vi "main(Test DQMH modules).vi"() -> ()   [LabVIEW 2018, in "Application.lvlib"] (continued)
      tunnel: w245 -> [w281 _ _ _ w1278 w1403 _ w1480 _ _ _ _ _ _ _ _ _ _ _ _ _ _ _ _ _ _ _ _ _ _ _ _ _ _ _ _ _ _ _ _ _ _ _ _ w2433 _ _ _ _ _ _ _ _ _ _ _ _ _ _ _ _ _ _ _ _ _ _ _ _ _ _ _ _ _ _ _ _ _ _ _ _ _ _ _ _ _ _ _ _ _ _ _ _ _ _ _ _ _ _ _ _ _ _ _ _ _ _ _ _ _ _ _ _ _ _ _ _ _ _ _ _ _ _ _ _ _ _ _ _ _ _ _ _ _ _ _ _ _ _ _ _ _ _ _ _ _ _ _ _ _ _ _ _ _ _ _ _ _ _ _ _ _ _ _ _ _ w9912 w10010 w10108 w10208 w10305 w10404 w10503 w10602 w10701 w10800 w10899 w10998 w11097 w11196 w11295 w11394 w11493 w11592 w11691 w11790 w11889 w11988 w12087 w12186 w12285 w12384 w12483 w12582 w12681 w12780 w12879 w12978 w13077 w13176 w13275 w13374 w13473 w13572 w13671 w13770 w13869 w13968 w14067 w14166 w14265 w14364 w14463 w14562 w14661 w14760 w14859 w14958 w15057 w15156 w15255 w15354 w15453 w15552 w15651 w15750]
      tunnel: [w274 w1237 w1249 w1259 w1277 w1409 w1450 w1490 w1515 w1531 w1542 w1553 w1568 w1583 w1598 w1613 w1627 w1651 w1680 w1710 w1766 w1803 w1825 w1848 w1870 w1903 w1921 w1939 w1957 w1989 w2017 w2042 w2070 w2103 w2122 w2144 w2177 w2194 w2219 w2247 w2279 w2309 w2354 w2387 w2432 w2497 w2573 w2648 w2723 w2798 w2873 w2934 w3037 w3113 w3187 w3271 w3353 w3435 w3517 w3599 w3681 w3763 w3845 w3927 w4009 w4091 w4174 w4257 w4340 w4423 w4506 w4571 w4690 w4773 w4856 w4939 w5023 w5107 w5191 w5275 w5359 w5443 w5527 w5611 w5695 w5779 w5864 w5949 w6034 w6119 w6204 w6289 w6374 w6459 w6544 w6629 w6715 w6801 w6887 w6973 w7059 w7145 w7231 w7317 w7403 w7449 w7491 w7531 w7572 w7613 w7654 w7695 w7736 w7777 w7818 w7859 w7900 w7941 w7982 w8023 w8065 w8105 w8146 w8187 w8228 w8270 w8310 w8352 w8392 w8433 w8475 w8515 w8556 w8597 w8638 w8679 w8720 w8761 w8803 w8843 w8884 w8925 w8967 w9008 w9048 w9089 w9130 w9171 w9212 w9253 w9294 w9335 w9376 w9417 w9458 w9499 w9540 w9581 w9622 w9663 w9704 w9745 w9786 w9827 w9868 w9903 1 ("DUT channel (1-11)") 1 ("DUT channel (1-11)") 1 ("DUT channel (1-11)") 1 ("DUT channel (1-11)") 1 ("DUT channel (1-11)") 1 ("DUT channel (1-11)") 2 ("DUT channel (1-11)") 2 ("DUT channel (1-11)") 2 ("DUT channel (1-11)") 2 ("DUT channel (1-11)") 2 ("DUT channel (1-11)") 2 ("DUT channel (1-11)") 3 ("DUT channel (1-11)") 3 ("DUT channel (1-11)") 3 ("DUT channel (1-11)") 3 ("DUT channel (1-11)") 3 ("DUT channel (1-11)") 3 ("DUT channel (1-11)") 4 ("DUT channel (1-11)") 4 ("DUT channel (1-11)") 4 ("DUT channel (1-11)") 4 ("DUT channel (1-11)") 4 ("DUT channel (1-11)") 4 ("DUT channel (1-11)") 5 ("DUT channel (1-11)") 5 ("DUT channel (1-11)") 5 ("DUT channel (1-11)") 5 ("DUT channel (1-11)") 5 ("DUT channel (1-11)") 5 ("DUT channel (1-11)") 6 ("DUT channel (1-11)") 6 ("DUT channel (1-11)") 6 ("DUT channel (1-11)") 6 ("DUT channel (1-11)") 6 ("DUT channel (1-11)") 6 ("DUT channel (1-11)") 7 ("DUT channel (1-11)") 7 ("DUT channel (1-11)") 7 ("DUT channel (1-11)") 7 ("DUT channel (1-11)") 7 ("DUT channel (1-11)") 7 ("DUT channel (1-11)") 8 ("DUT channel (1-11)") 8 ("DUT channel (1-11)") 8 ("DUT channel (1-11)") 8 ("DUT channel (1-11)") 8 ("DUT channel (1-11)") 8 ("DUT channel (1-11)") 9 ("DUT channel (1-11)") 9 ("DUT channel (1-11)") 9 ("DUT channel (1-11)") 9 ("DUT channel (1-11)") 9 ("DUT channel (1-11)") 9 ("DUT channel (1-11)") 10 ("DUT channel (1-11)") 10 ("DUT channel (1-11)") 10 ("DUT channel (1-11)") 10 ("DUT channel (1-11)") 10 ("DUT channel (1-11)") 10 ("DUT channel (1-11)")] -> w244
      tunnel: w243 -> [w275 w1237 w1249 w1259 w1277 w1409 w1450 w1490 w1515 w1531 w1542 w1553 w1568 w1583 w1598 w1613 w1627 w1651 w1680 w1710 w1766 w1803 w1825 w1848 w1870 w1903 w1921 w1939 w1957 w1989 w2017 w2042 w2070 w2103 w2122 w2144 w2177 w2194 w2219 w2247 w2279 w2309 w2354 w2387 w2432 _ _ _ _ _ _ _ _ _ _ _ _ _ _ _ _ _ _ _ _ _ _ _ _ _ _ _ _ _ _ _ _ _ _ _ _ _ _ _ _ _ _ _ _ _ _ _ _ _ _ _ _ _ _ _ _ _ _ _ _ w7449 w7491 w7531 w7572 w7613 w7654 w7695 w7736 w7777 w7818 w7859 w7900 w7941 w7982 w8023 w8065 w8105 w8146 w8187 w8228 w8270 w8310 w8352 w8392 w8433 w8475 w8515 w8556 w8597 w8638 w8679 w8720 w8761 w8803 w8843 w8884 w8925 w8967 w9008 w9048 w9089 w9130 w9171 w9212 w9253 w9294 w9335 w9376 w9417 w9458 w9499 w9540 w9581 w9622 w9663 w9704 w9745 w9786 w9827 w9868 w9903 _ _ _ _ _ _ _ _ _ _ _ _ _ _ _ _ _ _ _ _ _ _ _ _ _ _ _ _ _ _ _ _ _ _ _ _ _ _ _ _ _ _ _ _ _ _ _ _ _ _ _ _ _ _ _ _ _ _ _ _]
      tunnel: [w272 w1236 w1248 w1258 w1279 w1397 w1449 w1489 w1514 w1530 w1541 w1552 w1567 w1582 w1597 w1612 w1626 w1650 w1679 w1709 w1765 w1802 w1824 w1847 w1869 w1902 w1920 w1938 w1956 w1988 w2016 w2041 w2069 w2102 w2121 w2143 w2176 w2193 w2218 w2250 w2278 w2308 w2353 w2378 w2431 w2481 w2572 w2647 w2722 w2797 w2872 w2933 w3036 w3112 w3186 w3270 w3352 w3434 w3516 w3598 w3680 w3762 w3844 w3926 w4008 w4090 w4173 w4256 w4339 w4422 w4505 w4570 w4689 w4772 w4855 w4938 w5022 w5106 w5190 w5274 w5358 w5442 w5526 w5610 w5694 w5778 w5863 w5948 w6033 w6118 w6203 w6288 w6373 w6458 w6543 w6628 w6714 w6800 w6886 w6972 w7058 w7144 w7230 w7316 w7402 w7445 w7487 w7527 w7568 w7609 w7653 w7691 w7732 w7773 w7814 w7855 w7896 w7937 w7978 w8019 w8061 w8101 w8145 w8183 w8224 w8266 w8306 w8348 w8388 w8429 w8471 w8511 w8552 w8593 w8634 w8675 w8716 w8757 w8799 w8839 w8880 w8921 w8963 w9004 w9044 w9085 w9126 w9167 w9208 w9249 w9290 w9331 w9372 w9413 w9454 w9495 w9536 w9577 w9618 w9660 w9700 w9741 w9782 w9823 w9864 w9902 w9911 w10009 w10107 w10207 w10304 w10403 w10502 w10601 w10700 w10799 w10898 w10997 w11096 w11195 w11294 w11393 w11492 w11591 w11690 w11789 w11888 w11987 w12086 w12185 w12284 w12383 w12482 w12581 w12680 w12779 w12878 w12977 w13076 w13175 w13274 w13373 w13472 w13571 w13670 w13769 w13868 w13967 w14066 w14165 w14264 w14363 w14462 w14561 w14660 w14759 w14858 w14957 w15056 w15155 w15254 w15353 w15452 w15551 w15650 w15749] -> w242
      tunnel: w241 -> [w273 w1236 w1248 w1258 w1279 w1397 w1449 w1489 w1514 w1530 w1541 w1552 w1567 w1582 w1597 w1612 w1626 w1650 w1679 w1709 w1765 w1802 w1824 w1847 w1869 w1902 w1920 w1938 w1956 w1988 w2016 w2041 w2069 w2102 w2121 w2143 w2176 w2193 w2218 w2250 w2278 w2308 w2353 w2378 w2431 w2481 w2572 w2647 w2722 w2797 w2872 w2933 w3036 w3112 w3186 w3270 w3352 w3434 w3516 w3598 w3680 w3762 w3844 w3926 w4008 w4090 w4173 w4256 w4339 w4422 w4505 w4570 w4689 w4772 w4855 w4938 w5022 w5106 w5190 w5274 w5358 w5442 w5526 w5610 w5694 w5778 w5863 w5948 w6033 w6118 w6203 w6288 w6373 w6458 w6543 w6628 w6714 w6800 w6886 w6972 w7058 w7144 w7230 w7316 w7402 _ _ _ _ _ _ _ _ _ _ _ _ _ _ _ _ _ _ _ _ _ _ _ _ _ _ _ _ _ _ _ _ _ _ _ _ _ _ _ _ _ _ _ _ _ _ _ _ _ _ _ _ _ _ _ _ _ _ _ _ w9902 _ _ _ _ _ _ _ _ _ _ _ _ _ _ _ _ _ _ _ _ _ _ _ _ _ _ _ _ _ _ _ _ _ _ _ _ _ _ _ _ _ _ _ _ _ _ _ _ _ _ _ _ _ _ _ _ _ _ _ _]
      tunnel: w238 -> [w280 _ _ _ _ _ _ _ _ _ _ _ _ _ _ _ _ _ _ _ _ _ _ _ _ _ _ _ _ _ _ _ _ w2097 _ _ _ _ _ _ _ _ _ _ _ _ _ _ _ _ _ _ _ _ _ _ _ _ _ _ _ _ _ _ _ _ _ _ _ _ _ _ _ _ _ _ _ _ _ _ _ _ _ _ _ _ _ _ _ _ _ _ _ _ _ _ _ _ _ _ _ _ _ _ _ _ _ _ _ _ _ _ _ _ _ _ _ _ _ _ _ _ _ _ _ _ _ _ _ _ _ _ _ _ _ _ _ _ _ _ _ _ _ _ _ _ _ _ _ _ _ _ _ _ _ _ _ _ _ _ _ _ _ _ _ _ _ _ _ _ _ _ _ _ _ _ _ _ _ _ _ _ _ _ _ _ _ _ _ _ _ _ _ _ _ _ _ _ _ _ _ _ _ _ _ _ _ _ _ _ _ _ _ _ _ _ _ _ _ _ _ _ _ _ _ _]
      tunnel: [_ _ _ _ _ _ _ _ _ _ _ _ _ _ _ _ _ _ _ _ _ _ _ _ _ _ _ _ _ _ _ _ _ _ _ _ _ _ _ _ _ _ _ TRUE _ _ _ _ _ _ _ _ _ _ _ _ _ _ _ _ _ _ _ _ _ _ _ _ _ _ _ _ _ _ _ _ _ _ _ _ _ _ _ _ _ _ _ _ _ _ _ _ _ _ _ _ _ _ _ _ _ _ _ _ _ _ _ _ _ _ _ _ _ _ _ _ _ _ _ _ _ _ _ _ _ _ _ _ _ _ _ _ _ _ _ _ _ _ _ _ _ _ _ _ _ _ _ _ _ _ _ _ _ _ _ _ _ _ _ _ _ _ _ _ _ _ _ _ _ _ _ _ _ _ _ _ _ _ _ _ _ _ _ _ _ _ _ _ _ _ _ _ _ _ _ _ _ _ _ _ _ _ _ _ _ _ _ _ _ _ _ _ _ _ _ _ _ _ _ _ _ _ _ _ _ _] -> w237
      tunnel: [w276 "Waiting for JIG lock" w1242 w1254 w1275 w1407 w1422 w1481 w1513 w1529 w1540 w1551 w1566 w1581 w1596 w1611 w1624 w1646 w1678 "Initialize Apps" w1747 w1798 w1820 w1843 w1864 w1897 w1915 w1933 w1951 w1978 w2011 w2038 w2066 w2093 "HV-60D ready!!!!!!!!!!!!!!!!" w2138 w2173 w2188 w2211 w2244 w2274 w2303 w2346 w2380 "Shorted Circuit Test" "Test Channel 1" "Test Channel 2" "Test Channel 3" "Test Channel 4" "Test Channel 5" "Test Channel 6" "Test Channel 7" "Test Channel 8" "Test Channel 9" "Test Channel 10" "Test Channel 10A" "Test Channel 1A" "Test Channel 2A" "Test Channel 3A" "Test Channel 4A" "Test Channel 5A" "Test Channel 6A" "Test Channel 7A" "Test Channel 8A" "Test Channel 9A" "Test Channel 10B" "Test Channel 1B" "Test Channel 2B" "Test Channel 3B" "Test Channel 4B" "Test Channel 5B" "Test Channel 6B" "Test Channel 7B" "Test Channel 8B" "Test Channel 9B" "Test Channel 10C" "Test Channel 1C" "Test Channel 2C" "Test Channel 3C" "Test Channel 4C" "Test Channel 5C" "Test Channel 6C" "Test Channel 7C" "Test Channel 8C" "Test Channel 9C" "Test Channel 10D" "Test Channel 1D" "Test Channel 2D" "Test Channel 3D" "Test Channel 4D" "Test Channel 5D" "Test Channel 6D" "Test Channel 7D" "Test Channel 8D" "Test Channel 9D" "Test Channel 10E" "Test Channel 1E" "Test Channel 2E" "Test Channel 3E" "Test Channel 4E" "Test Channel 5E" "Test Channel 6E" "Test Channel 7E" "Test Channel 8E" "Test Channel 9E" w7447 w7490 w7530 w7571 w7612 w7652 w7694 w7735 w7776 w7817 w7858 w7899 w7940 w7981 w8022 w8064 w8104 w8144 w8186 w8227 w8269 w8309 w8351 w8391 w8432 w8474 w8514 w8555 w8596 w8637 w8678 w8719 w8760 w8802 w8842 w8883 w8924 w8966 w9007 w9047 w9088 w9129 w9170 w9211 w9252 w9293 w9334 w9375 w9416 w9457 w9498 w9539 w9580 w9621 w9662 w9703 w9744 w9785 w9826 w9867 w9901 w9916 w10014 w10112 w10210 w10309 w10408 w10507 w10606 w10705 w10804 w10903 w11002 w11101 w11200 w11299 w11398 w11497 w11596 w11695 w11794 w11893 w11992 w12091 w12190 w12289 w12388 w12487 w12586 w12685 w12784 w12883 w12982 w13081 w13180 w13279 w13378 w13477 w13576 w13675 w13774 w13873 w13972 w14071 w14170 w14269 w14368 w14467 w14566 w14665 w14764 w14863 w14962 w15061 w15160 w15259 w15358 w15457 w15556 w15655 w15754] -> w234
      tunnel: w233 -> [w277 _ w1242 w1254 w1275 w1407 _ _ w1513 w1529 w1540 w1551 w1566 w1581 w1596 w1611 w1624 w1646 w1678 _ w1746 w1798 w1820 w1843 w1864 w1897 w1915 w1933 w1951 w1978 w2011 w2038 w2066 w2093 _ w2138 w2173 w2188 w2211 w2244 w2274 w2303 w2346 w2380 _ _ _ _ _ _ _ _ _ _ _ _ _ _ _ _ _ _ _ _ _ _ _ _ _ _ _ _ _ _ _ _ _ _ _ _ _ _ _ _ _ _ _ _ _ _ _ _ _ _ _ _ _ _ _ _ _ _ _ _ _ w7446 w7489 w7529 w7570 w7611 w7651 w7693 w7734 w7775 w7816 w7857 w7898 w7939 w7980 w8021 w8063 w8103 w8143 w8185 w8226 w8268 w8308 w8350 w8390 w8431 w8473 w8513 w8554 w8595 w8636 w8677 w8718 w8759 w8801 w8841 w8882 w8923 w8965 w9006 w9046 w9087 w9128 w9169 w9210 w9251 w9292 w9333 w9374 w9415 w9456 w9497 w9538 w9579 w9620 w9661 w9702 w9743 w9784 w9825 w9866 w9901 _ _ _ _ _ _ _ _ _ _ _ _ _ _ _ _ _ _ _ _ _ _ _ _ _ _ _ _ _ _ _ _ _ _ _ _ _ _ _ _ _ _ _ _ _ _ _ _ _ _ _ _ _ _ _ _ _ _ _ _]
      tunnel: w231 -> [_ _ _ _ _ _ w1430 _ _ _ _ _ _ _ _ _ _ _ _ _ _ _ _ _ _ _ _ _ _ _ _ _ _ _ _ _ _ _ _ _ _ _ _ _ _ _ _ _ _ _ _ _ _ _ _ _ _ _ _ _ _ _ _ _ _ _ _ _ _ _ _ _ _ _ _ _ _ _ _ _ _ _ _ _ _ _ _ _ _ _ _ _ _ _ _ _ _ _ _ _ _ _ _ _ _ _ _ _ _ _ _ _ _ _ _ _ _ _ _ _ _ _ _ _ _ _ _ _ _ _ _ _ _ _ _ _ _ _ _ _ _ _ _ _ _ _ _ _ _ _ _ _ _ _ _ _ _ _ _ _ _ _ _ _ _ _ _ _ _ _ _ _ _ _ _ _ _ _ _ _ _ _ _ _ _ _ _ _ _ _ _ _ _ _ _ _ _ _ _ _ _ _ _ _ _ _ _ _ _ _ _ _ _ _ _ _ _ _ _ _ _ _ _ _ _ _]
      frame "Apps.WaitForEvent", Default {
        n145 = event shown="[38] \"Test Channel 10\": Value Change" {
          selector: w289 -> [_ w316 _ _ _ _ _ _ _ _ _ _ _ _ _ _ _ _ _ _ _ _ _ _ _ _ _ _ _ _ _ _ _ _ _ _ _ _ _ _ _ _]
          dyn-events: [_ w316 _ _ _ _ _ _ _ _ _ _ _ _ _ _ _ _ _ _ _ _ _ _ _ _ _ _ _ _ _ _ _ _ _ _ _ _ _ _ _ _] -> w288
          timeout: w278 -> [_ _ _ _ _ _ _ _ _ _ _ _ _ _ _ _ _ _ _ _ _ _ _ _ _ _ _ _ _ _ _ _ _ _ _ _ _ _ _ _ _ _]
          tunnel: [w297 w311 w328 w350 w369 w386 w398 w430 w441 w459 w467 w488 w506 w522 w534 w554 w575 w609 w627 w643 w667 w685 w703 w731 w770 w789 w817 w924 w953 w976 w997 w1018 w1039 w1060 w1081 w1102 w1123 w1144 w1165 w1180 w1200 w1223] -> w290
          tunnel: w278 -> [w297 w311 w329 w350 w369 w386 w398 w430 w441 w459 w467 w488 w506 w522 w534 w554 w575 w609 w627 w643 w667 w685 w703 w731 w770 w789 w817 w924 w953 w976 w997 w1018 w1039 w1060 w1081 w1102 w1123 w1144 w1165 w1180 w1200 w1223]
          tunnel: [w291 w315 w326 w339 w359 w383 w390 w424 w435 w449 w465 w483 w496 w514 w530 w552 w573 w602 w622 w640 w665 w683 w701 w725 w762 w783 w813 w923 w950 w974 w995 w1016 w1037 w1058 w1079 w1100 w1121 w1142 w1163 w1171 w1197 w1214] -> w286
          tunnel: w285 -> [w295 w315 w326 w343 w358 w385 w409 w425 w437 w458 w464 w482 w501 w515 w529 w551 w572 w601 w621 w639 w664 w682 w700 w724 w764 w787 w812 w922 w951 w975 w996 w1017 w1038 w1059 w1080 w1101 w1122 w1143 w1164 w1171 w1196 w1214]
          tunnel: w284 -> [w298 w309 w330 w345 _ w374 w411 w428 w438 w457 w470 w487 w505 _ w524 w559 w579 w606 w626 w651 w670 w688 w708 w728 w769 w790 w814 w912 w947 w971 w992 w1013 w1034 w1055 w1076 w1098 w1118 w1139 w1160 w1173 w1191 w1216]
          tunnel: [w301 w318 w334 w349 w368 w382 w410 w429 w439 w453 w466 w485 w502 w521 w531 w553 w574 w603 w623 w642 w666 w684 w702 w730 w765 w784 w815 w925 w946 w969 w990 w1011 w1032 w1053 w1074 w1096 w1116 w1137 w1158 w1179 w1199 w1222] -> w283
          tunnel: w282 -> [w301 w318 w334 w349 w368 w382 w410 w429 w439 w453 w466 w485 w502 w521 w531 w553 w574 w603 w623 w642 w666 w684 w702 w730 w765 _ w816 w925 w946 w969 w990 w1011 w1032 w1053 w1074 w1096 w1116 w1137 w1158 w1179 w1199 w1222]
          tunnel: w281 -> [_ _ _ w340 _ _ w400 _ _ _ _ _ _ _ _ _ _ _ _ _ _ _ _ _ _ _ _ _ _ w968 w987 w1007 w1028 w1049 w1070 w1091 w1112 w1133 w1154 _ _ _]
          tunnel: w279 -> [w300 w317 _ _ _ _ _ _ _ _ w463 w481 w500 _ w528 w550 w571 w600 w620 w638 w663 w681 w699 w723 w761 w785 w810 w921 _ _ _ _ _ _ _ _ _ _ _ w1178 w1198 w1221]
          tunnel: w280 -> [_ _ _ _ _ _ _ _ _ _ _ _ _ _ _ _ _ _ _ _ _ _ _ _ _ _ _ _ _ _ _ _ _ _ _ _ _ _ _ _ _ _]
          tunnel: w275 -> [w293 w313 w333 w347 w366 w380 w402 w422 w433 w451 w461 w479 w498 w519 w526 w548 _ w598 w618 w636 w661 w679 w697 w720 w759 w779 w807 w908 w944 _ _ _ _ _ _ _ _ _ _ w1176 w1194 w1219]
          tunnel: w277 -> [w294 _ _ w348 w367 w381 _ _ w434 w452 w462 w480 w499 w520 w527 w549 w570 w599 w619 w637 w662 w680 w698 w722 w760 w780 w808 w909 w945 w964 w985 w1006 w1027 w1048 w1069 w1090 w1111 w1132 w1153 w1177 w1195 w1220]
          tunnel: [w294 "Waiting for JIG lock" "Waiting for JIG lock" w348 w367 w381 "Start Auto Test" "Settings" w434 w452 w462 w480 w499 w520 w527 w549 w570 w599 w619 w637 w662 w680 w698 w722 w760 w780 w808 w909 w945 w964 w985 w1006 w1027 w1048 w1069 w1090 w1111 w1132 w1153 w1177 w1195 w1220] -> w276
          tunnel: [w293 w313 w333 w347 w366 w380 w402 w422 w433 w451 w461 w479 w498 w519 w526 w548 w567 w598 w618 w636 w661 w679 w697 w720 w759 w779 w806 w908 w944 1 ("DUT channel (1-11)") 2 ("DUT channel (1-11)") 3 ("DUT channel (1-11)") 4 ("DUT channel (1-11)") 5 ("DUT channel (1-11)") 6 ("DUT channel (1-11)") 7 ("DUT channel (1-11)") 8 ("DUT channel (1-11)") 9 ("DUT channel (1-11)") 10 ("DUT channel (1-11)") w1176 w1194 w1219] -> w274
          tunnel: w273 -> [w292 w312 w332 w346 w365 w379 w401 w421 w432 w450 w460 w478 w497 w518 w525 w547 w569 w597 w617 w635 w660 w678 w696 _ w758 w778 w802 w907 w943 w962 w983 w1004 w1025 w1046 w1067 w1088 w1109 w1130 w1151 w1172 w1190 w1215]
          tunnel: [w292 w312 w332 w346 w365 w379 w401 w421 w432 w450 w460 w478 w497 w518 w525 w547 w569 w597 w617 w635 w660 w678 w696 w716 w758 w778 w801 w907 w943 w962 w983 w1004 w1025 w1046 w1067 w1088 w1109 w1130 w1151 w1172 w1190 w1215] -> w272
          tunnel: w271 -> [_ _ _ _ _ _ _ _ _ _ _ _ _ _ _ _ _ _ _ _ _ _ _ _ _ _ w805 _ _ _ _ _ _ _ _ _ _ _ _ _ _ _]
          event Timeout {
            n146 = event-data() -> ()  [unwired: 1 in, 1 out]
            n147 = disable-structure shown="LOGGING==TRUE" {
              disable-tunnel: w300 -> [w302 _]
              frame condition #0 (active) {
                n148 = Empty String/Path?(string/path=w302) -> (empty?=w308:bool)
                n149 = Select(t="Quece timeout", s=w308, f=w302) -> (s? t:f=w306:string)
                n150 = Format Into String(format string=": %s", initial string=w306, "UI timeout") -> (resulting string=w303:string)  [unwired: 1 in, 1 out]
                n151 = call "string log (SubVI).vi"("state Name"=w303) -> ()  [unwired: 9 in, 2 out]
              }
              frame condition #1 {
              }
            }
            n152 = call "App enquece.vi"("command"="Apps.WaitingForTrigger", "queue in"=w298) -> ("error out"=w296:errorcluster)  [unwired: 8 in, 1 out]
            n153 = Merge Errors(w295, w296) -> (w291:errorcluster)
          }
          event "Test": Value Change {
            n154 = event-data() -> ()  [unwired: 1 in, 1 out]
            n155 = disable-structure shown="LOGGING==TRUE" {
              disable-tunnel: w317 -> [w319 _]
              frame condition #0 (active) {
                n156 = Empty String/Path?(string/path=w319) -> (empty?=w325:bool)
                n157 = Select(t="Quece timeout", s=w325, f=w319) -> (s? t:f=w323:string)
                n158 = Format Into String(format string=": %s", initial string=w323, "Test") -> (resulting string=w320:string)  [unwired: 1 in, 1 out]
                n159 = call "string log (SubVI).vi"("state Name"=w320) -> ()  [unwired: 9 in, 2 out]
              }
              frame condition #1 {
              }
            }
            n160 = call "App enquece.vi"("command"="Apps.AutoMode", "queue in"=w309) -> ()  [unwired: 8 in, 2 out]
          }
          event "Auto/Man": Value Change {
            n161 = event-data() -> ("NewVal"=w331:bool)  [unwired: 1 in]
            n162 = case shown="True" w331 {
              tunnel: w330 -> [_ w337]
              tunnel: [-1 w336] -> w328
              tunnel: w329 -> [_ w336]
              frame False {
              }
              frame True {
                n163 = call "App enquece.vi"("command"="Apps.AutoMode", "queue in"=w337) -> ()  [unwired: 8 in, 2 out]
              }
            }
          }
          event "Test Single DRV": Value Change {
            n164 = event-data() -> ()  [unwired: 1 in, 1 out]
            n165 = case shown="1.." "DRV number" {
              selector: "DRV number" -> [_ w353]
              tunnel: ["MEAS.AllRelaysOFF" w356] -> w344
              tunnel: w340 -> [w351 _]
              frame 0, Default {
                n166 = call "reset DRV UI (SubVI).vi"("Ref  in"=w351) -> ()  [unwired: 9 in, 2 out]
              }
              frame 1.. {
                n167 = Format Into String(format string="%d%s", initial string="Test DRV ", w353, "A" ("input 3")) -> (resulting string=w356:string)  [unwired: 1 in, 1 out]
              }
            }
            n168 = call "App enquece.vi"("command"=w344, "queue in"=w345) -> ("error out"=w342:errorcluster)  [unwired: 8 in, 1 out]
            n169 = Merge Errors(w343, w342) -> (w339:errorcluster)
          }
          event "DMM query": Value Change {
            n170 = event-data() -> ()  [unwired: 1 in, 1 out]
            n171 = flat-sequence {
              tunnel: [w370] -> w363
              frame #0 {
                w371 = ""
                n172 = Wait (ms)(milliseconds to wait=u32 100) -> ()  [unwired: 1 out]
                n173 = local write "DMM func?"(w371) -> ()
                n174 = local write "DMM range?"(w371) -> ()
                n175 = xnode "Error Ring"() -> ("error out"=w370:errorcluster)
              }
            }
            n176 = call "Query func.vi"("error in"=w363) -> ("error out"=w361:errorcluster, "String"=→"DMM func?":string)  [unwired: 8 in, 1 out]
            n177 = call "query range.vi"("error in"=w361) -> ("error out"=w360:errorcluster, "String"=→"DMM range?":string)  [unwired: 8 in, 1 out]
            n178 = Merge Errors(w358, w360) -> (w359:errorcluster)
          }
          event "VIEW": Value Change {
            n179 = event-data() -> ()  [unwired: 1 in, 1 out]
            n180 = disable-structure shown="Disabled" {
              disable-tunnel: w374 -> [w388 _]
              frame Disabled {
                n181 = call "App enquece.vi"("command"="Apps.UI Update 1", "queue in"=w388) -> ()  [unwired: 8 in, 2 out]
              }
              frame Enabled {
              }
            }
            n182 = invoke class="VI" method="FP.Open"("State"=T17."Hidden") -> (error out=w378:errorcluster)  [unwired: 4 in, 4 out]
            n183 = call "View DRV data.vi"("error in (no error)"=w378) -> ("error out"=w377:errorcluster)  [unwired: 10 in]
            n184 = invoke class="VI" method="FP.Open"(error in=w377, "State"=T17."Standard") -> (error out=w384:errorcluster)  [unwired: 3 in, 4 out]
            n185 = Merge Errors(w385, w384) -> (w383:errorcluster)
          }
          event User Event {
            # "#HungNotes:\nStart HV60D from this frame (check new board  installed)"
            n186 = event-data() -> ("new board?"=w406:bool, "new trigger"=→"new Trigger?":bool, "last trigger"=→"last Trigger?":bool)  [unwired: 1 in]
            "New board?" <- w406
            n187 = call "reset DRV UI (SubVI).vi"("Ref  in"=w400) -> ()  [unwired: 9 in, 2 out]
            n188 = case shown="True" w406 {
              tunnel: w411 -> [_ w417]
              tunnel: [_ w416] -> w397
              frame False {
              }
              frame True {
                n189 = call "FGV DUT steps.vi"("Enum(read)"=enum16{"write", "read"}."read" ("Enum")) -> ("Steps OUT"=w414:string[])  [unwired: 10 in]
                n190 = Array Subset(array=w414, index=3) -> (w412:string[])  [unwired: 1 in]
                n191 = for {
                  tunnel: [w420] -> w416 mode=indexing
                  tunnel: w417 -> [w419]
                  tunnel: w412 -> [w418] mode=indexing
                  n192 = call "App enquece.vi"("command"=w418, "queue in"=w419) -> ("error out"=w420:errorcluster)  [unwired: 8 in, 1 out]
                }
              }
            }
            n193 = control-ref of="DRV 61"() -> (w404:refnum<vi>)
            n194 = Merge Errors(w397) -> (w396:errorcluster)
            n195 = property class="ColBox"(reference=w404, error in=w396, "Value"=u32 10000536 ("DRV 1")) -> (error out=w395:errorcluster)  [unwired: 1 out]
            n196 = local write "Report file Name"("") -> ()
            n197 = Merge Errors(w409, w395) -> (w394:errorcluster)
            n198 = call "string log (SubVI).vi"("Enum(log)"=enum16{"Init", "Log", "Read", "Clear"}."Clear") -> ("error out"=w391:errorcluster)  [unwired: 9 in, 1 out]
            n199 = call "FGV Driver Data.vi"("error in (no error)"=w391, "FGV enum(Read)"=FGV_DRV_data."Init") -> ("error out"=w389:errorcluster)  [unwired: 6 in, 3 out]
            n200 = Merge Errors(w394, w389) -> (w390:errorcluster)
          }
          event "Settings": Value Change {
            n201 = event-data() -> ()  [unwired: 1 in, 1 out]
            n202 = call "App enquece.vi"("command"="INIT.Read DRV code", "queue in"=w428) -> ("error out"=w426:errorcluster)  [unwired: 8 in, 1 out]
            n203 = Merge Errors(w425, w426) -> (w424:errorcluster)
          }
          event Panel Close? {
            n204 = event-data() -> ()  [unwired: 1 in, 1 out]
            n205 = disable-structure shown="Enabled" {
              disable-tunnel: [w442 TRUE] -> w431
              frame Enabled {
                n206 = Two Button Dialog(message="Do you want to exit progam") -> (T button?=w442:bool)  [unwired: 2 in]
              }
              frame Disabled {
              }
            }
            n207 = case shown="True" w431 {
              tunnel: w438 -> [_ w447]
              tunnel: [_ w445] -> w436
              frame False {
              }
              frame True {
                n208 = call "App enquece.vi"("Priority Enquece"=TRUE, "command"="Apps.Exit", "queue in"=w447) -> ("error out"=w445:errorcluster)  [unwired: 7 in, 1 out]
              }
            }
            n209 = Merge Errors(w437, w436) -> (w435:errorcluster)
            n210 = event-data("Discard?"=TRUE) -> ()  [unwired: 1 in, 1 out]
          }
          event "Exit": Value Change {
            n211 = event-data() -> ()  [unwired: 1 in, 1 out]
            n212 = call "App enquece.vi"("Priority Enquece"=TRUE, "command"="Apps.Exit", "queue in"=w457) -> ("error out"=w456:errorcluster)  [unwired: 7 in, 1 out]
            n213 = Merge Errors(w458, w456) -> (w449:errorcluster)
          }
          event "check connected": Value Change {
            n214 = event-data() -> ()  [unwired: 1 in, 1 out]
            n215 = disable-structure shown="LOGGING==TRUE" {
              disable-tunnel: w463 -> [w471 _]
              frame condition #0 (active) {
                n216 = Empty String/Path?(string/path=w471) -> (empty?=w477:bool)
                n217 = Select(t="Quece timeout", s=w477, f=w471) -> (s? t:f=w475:string)
                n218 = Format Into String(format string=": %s", initial string=w475, "Check connected") -> (resulting string=w472:string)  [unwired: 1 in, 1 out]
                n219 = call "string log (SubVI).vi"("state Name"=w472) -> ()  [unwired: 9 in, 2 out]
              }
              frame condition #1 {
              }
            }
            n220 = call "App enquece.vi"("command"="MEAS.Read EMIC connected", "queue in"=w470) -> ("error out"=w468:errorcluster)  [unwired: 8 in, 1 out]
            n221 = Merge Errors(w464, w468) -> (w465:errorcluster)
          }
          event "Open COM eMIC": Value Change {
            n222 = event-data() -> ()  [unwired: 1 in, 1 out]
            n223 = disable-structure shown="LOGGING==TRUE" {
              disable-tunnel: w481 -> [w489 _]
              frame condition #0 (active) {
                n224 = Empty String/Path?(string/path=w489) -> (empty?=w495:bool)
                n225 = Select(t="Quece timeout", s=w495, f=w489) -> (s? t:f=w493:string)
                n226 = Format Into String(format string=": %s", initial string=w493, "Open COM eMIC") -> (resulting string=w490:string)  [unwired: 1 in, 1 out]
                n227 = call "string log (SubVI).vi"("state Name"=w490) -> ()  [unwired: 9 in, 2 out]
              }
              frame condition #1 {
              }
            }
            n228 = call "App enquece.vi"("command"="INIT.Open COM EMIC", "queue in"=w487) -> ("error out"=w486:errorcluster)  [unwired: 8 in, 1 out]
            n229 = Merge Errors(w482, w486) -> (w483:errorcluster)
          }
          event "Read trigger": Value Change {
            n230 = event-data() -> ()  [unwired: 1 in, 1 out]
            n231 = disable-structure shown="LOGGING==TRUE" {
              disable-tunnel: w500 -> [w507 _]
              frame condition #0 (active) {
                n232 = Empty String/Path?(string/path=w507) -> (empty?=w513:bool)
                n233 = Select(t="Quece timeout", s=w513, f=w507) -> (s? t:f=w511:string)
                n234 = Format Into String(format string=": %s", initial string=w511, "Read Trigger") -> (resulting string=w508:string)  [unwired: 1 in, 1 out]
                n235 = call "string log (SubVI).vi"("state Name"=w508) -> ()  [unwired: 9 in, 2 out]
              }
              frame condition #1 {
              }
            }
            n236 = call "App enquece.vi"("command"="MEAS.Read TRIGGER", "queue in"=w505) -> ("error out"=w503:errorcluster)  [unwired: 8 in, 1 out]
            n237 = Merge Errors(w501, w503) -> (w496:errorcluster)
          }
          event "Set trigger value": Value Change {
            n238 = event-data() -> ()  [unwired: 1 in, 6 out]
            n239 = call "SET trigger value.vi"("Boolean"="set value") -> ("error out"=w516:errorcluster)  [unwired: 10 in]
            n240 = Merge Errors(w515, w516) -> (w514:errorcluster)
          }
          event "Read Optos": Value Change {
            n241 = event-data() -> ()  [unwired: 1 in, 1 out]
            n242 = disable-structure shown="LOGGING==TRUE" {
              disable-tunnel: w528 -> [w540 _]
              frame condition #0 (active) {
                n243 = Empty String/Path?(string/path=w540) -> (empty?=w546:bool)
                n244 = Select(t="Quece timeout", s=w546, f=w540) -> (s? t:f=w544:string)
                n245 = Format Into String(format string=": %s", initial string=w544, "Read Optos") -> (resulting string=w541:string)  [unwired: 1 in, 1 out]
                n246 = call "string log (SubVI).vi"("state Name"=w541) -> ()  [unwired: 9 in, 2 out]
              }
              frame condition #1 {
              }
            }
            n247 = flat-sequence {
              tunnel: w524 -> [w535]
              tunnel: [w535] -> w523
              frame #0 {
                n248 = Initialize Array(FALSE, 6 ("dimension size"), 10 ("dimension size")) -> (w539:bool[][])
                n249 = local write "Short DRV"(w539) -> ()
              }
            }
            n250 = call "App enquece.vi"("command"="MEAS.Read Optos", "queue in"=w523) -> ("error out"=w532:errorcluster)  [unwired: 8 in, 1 out]
            n251 = Merge Errors(w529, w532) -> (w530:errorcluster)
          }
          event "Select DMM's Current Input": Value Change {
            n252 = event-data() -> ()  [unwired: 1 in, 1 out]
            n253 = disable-structure shown="LOGGING==TRUE" {
              disable-tunnel: w550 -> [w560 _]
              frame condition #0 (active) {
                n254 = Empty String/Path?(string/path=w560) -> (empty?=w566:bool)
                n255 = Select(t="Quece timeout", s=w566, f=w560) -> (s? t:f=w564:string)
                n256 = Format Into String(format string=": %s", initial string=w564, "DMM Current Input") -> (resulting string=w561:string)  [unwired: 1 in, 1 out]
                n257 = call "string log (SubVI).vi"("state Name"=w561) -> ()  [unwired: 9 in, 2 out]
              }
              frame condition #1 {
              }
            }
            n258 = To Variant(anything="mux2-1(DMM I) encode") -> (Variant=w556:variant)
            n259 = call "App enquece.vi"("command data"=w556, "command"="MEAS.Sel Input Current", "queue in"=w559) -> ("error out"=w555:errorcluster)  [unwired: 7 in, 1 out]
            n260 = Merge Errors(w551, w555) -> (w552:errorcluster)
          }
          event "DEMUX 1-10": Value Change {
            n261 = event-data() -> ()  [unwired: 1 in, 1 out]
            n262 = disable-structure shown="LOGGING==TRUE" {
              disable-tunnel: w571 -> [w590 _]
              frame condition #0 (active) {
                n263 = Empty String/Path?(string/path=w590) -> (empty?=w596:bool)
                n264 = Select(t="Quece timeout", s=w596, f=w590) -> (s? t:f=w594:string)
                n265 = Format Into String(format string=": %s", initial string=w594, "demux1-10") -> (resulting string=w591:string)  [unwired: 1 in, 1 out]
                n266 = call "string log (SubVI).vi"("state Name"=w591) -> ()  [unwired: 9 in, 2 out]
              }
              frame condition #1 {
              }
            }
            n267 = To Variant(anything="demux1_10(x6)_encode") -> (Variant=w577:variant)
            n268 = case shown="\"demux1_10_channel1\"" "demux1_10(x6)_encode" {
              tunnel: [_ 1 ("DUT channel (1-11)") 2 ("DUT channel (1-11)") 3 ("DUT channel (1-11)") 4 ("DUT channel (1-11)") 5 ("DUT channel (1-11)") 6 ("DUT channel (1-11)") 7 ("DUT channel (1-11)") 8 ("DUT channel (1-11)") 9 ("DUT channel (1-11)") 10 ("DUT channel (1-11)")] -> w567
              frame "demux1_10_channel0", Default {
              }
              frame "demux1_10_channel1" {
              }
              frame "demux1_10_channel2" {
              }
              frame "demux1_10_channel3" {
              }
              frame "demux1_10_channel4" {
              }
              frame "demux1_10_channel5" {
              }
              frame "demux1_10_channel6" {
              }
              frame "demux1_10_channel7" {
              }
              frame "demux1_10_channel8" {
              }
              frame "demux1_10_channel9" {
              }
              frame "demux1_10_channel10" {
              }
            }
            n269 = call "App enquece.vi"("command data"=w577, "command"="MEAS.demux1-10", "queue in"=w579) -> ("error out"=w576:errorcluster)  [unwired: 7 in, 1 out]
            n270 = Merge Errors(w572, w576) -> (w573:errorcluster)
          }
          event "eMIC": Value Change {
            n271 = event-data() -> ()  [unwired: 1 in, 1 out]
            n272 = disable-structure shown="LOGGING==TRUE" {
              disable-tunnel: w600 -> [w610 _]
              frame condition #0 (active) {
                n273 = Empty String/Path?(string/path=w610) -> (empty?=w616:bool)
                n274 = Select(t="Quece timeout", s=w616, f=w610) -> (s? t:f=w614:string)
                n275 = Format Into String(format string=": %s", initial string=w614, "eMIC") -> (resulting string=w611:string)  [unwired: 1 in, 1 out]
                n276 = call "string log (SubVI).vi"("state Name"=w611) -> ()  [unwired: 9 in, 2 out]
              }
              frame condition #1 {
              }
            }
            n277 = To Variant(anything="eMIC 6 values") -> (Variant=w604:variant)
            n278 = call "App enquece.vi"("command data"=w604, "command"="MEAS.eMIC", "queue in"=w606) -> ("error out"=w608:errorcluster)  [unwired: 7 in, 1 out]
            n279 = Merge Errors(w601, w608) -> (w602:errorcluster)
          }
          event "connect DMM": Value Change {
            n280 = event-data() -> ()  [unwired: 1 in, 1 out]
            n281 = disable-structure shown="LOGGING==TRUE" {
              disable-tunnel: w620 -> [w628 _]
              frame condition #0 (active) {
                n282 = Empty String/Path?(string/path=w628) -> (empty?=w634:bool)
                n283 = Select(t="Quece timeout", s=w634, f=w628) -> (s? t:f=w632:string)
                n284 = Format Into String(format string=": %s", initial string=w632, "Connect DMM") -> (resulting string=w629:string)  [unwired: 1 in, 1 out]
                n285 = call "string log (SubVI).vi"("state Name"=w629) -> ()  [unwired: 9 in, 2 out]
              }
              frame condition #1 {
              }
            }
            n286 = call "App enquece.vi"("command"="INIT.Open COM DMM", "queue in"=w626) -> ("error out"=w625:errorcluster)  [unwired: 8 in, 1 out]
            n287 = Merge Errors(w621, w625) -> (w622:errorcluster)
          }
          event "config DMM": Value Change {
            n288 = event-data() -> ()  [unwired: 1 in, 1 out]
            n289 = disable-structure shown="LOGGING==TRUE" {
              disable-tunnel: w638 -> [w652 _]
              frame condition #0 (active) {
                n290 = Empty String/Path?(string/path=w652) -> (empty?=w659:bool)
                n291 = Select(t="Quece timeout", s=w659, f=w652) -> (s? t:f=w657:string)
                n292 = Format Into String(format string=": %s", initial string=w657, "config DMM") -> (resulting string=w654:string)  [unwired: 1 in, 1 out]
                n293 = call "string log (SubVI).vi"("Enum(log)"=enum16{"Init", "Log", "Read"}."Log" ("Enum"), "state Name"=w654) -> ()  [unwired: 8 in, 2 out]
              }
              frame condition #1 {
              }
            }
            n294 = Bundle By Name(cluster=T19 {"DMM config cluster"={"DCV range"=0.0, "DCI range"=0.0, "Detector Rate"=0}, "mux2-1(DMM I) encode"=enum."DMM I (0.5)"} ("DMM all config"), "DMM config cluster.DCV range"="DCV range", "DMM config cluster.DCI range"="DCI range", "DMM config cluster.Detector Rate"="Detector Rate") -> (w646:T19)
            n295 = To Variant(anything=w646) -> (Variant=w644:variant)
            n296 = call "App enquece.vi"("command data"=w644, "command"="MEAS.Set DMM config", "queue in"=w651) -> ("error out"=w641:errorcluster)  [unwired: 7 in, 1 out]
            n297 = Merge Errors(w639, w641) -> (w640:errorcluster)
          }
          event "DMM read dual value": Value Change {
            n298 = event-data() -> ()  [unwired: 1 in, 1 out]
            n299 = disable-structure shown="LOGGING==TRUE" {
              disable-tunnel: w663 -> [w671 _]
              frame condition #0 (active) {
                n300 = Empty String/Path?(string/path=w671) -> (empty?=w677:bool)
                n301 = Select(t="Quece timeout", s=w677, f=w671) -> (s? t:f=w675:string)
                n302 = Format Into String(format string=": %s", initial string=w675, "DMM read dual value") -> (resulting string=w672:string)  [unwired: 1 in, 1 out]
                n303 = call "string log (SubVI).vi"("state Name"=w672) -> ()  [unwired: 9 in, 2 out]
              }
              frame condition #1 {
              }
            }
            n304 = call "App enquece.vi"("command"="MEAS.DMM dual read", "queue in"=w670) -> ("error out"=w668:errorcluster)  [unwired: 8 in, 1 out]
            n305 = Merge Errors(w664, w668) -> (w665:errorcluster)
          }
          event "Reset JIG": Value Change {
            n306 = event-data() -> ()  [unwired: 1 in, 1 out]
            n307 = disable-structure shown="LOGGING==TRUE" {
              disable-tunnel: w681 -> [w689 _]
              frame condition #0 (active) {
                n308 = Empty String/Path?(string/path=w689) -> (empty?=w695:bool)
                n309 = Select(t="Quece timeout", s=w695, f=w689) -> (s? t:f=w693:string)
                n310 = Format Into String(format string=": %s", initial string=w693, "reset JIG") -> (resulting string=w690:string)  [unwired: 1 in, 1 out]
                n311 = call "string log (SubVI).vi"("state Name"=w690) -> ()  [unwired: 9 in, 2 out]
              }
              frame condition #1 {
              }
            }
            n312 = call "App enquece.vi"("command"="MEAS.Reset JIG", "queue in"=w688) -> ("error out"=w686:errorcluster)  [unwired: 8 in, 1 out]
            n313 = Merge Errors(w682, w686) -> (w683:errorcluster)
          }
          event "TurnON/OFF +5V": Value Change {
            n314 = event-data() -> ()  [unwired: 1 in, 1 out]
            n315 = disable-structure shown="LOGGING==TRUE" {
              disable-tunnel: w699 -> [w709 _]
              frame condition #0 (active) {
                n316 = Empty String/Path?(string/path=w709) -> (empty?=w715:bool)
                n317 = Select(t="Quece timeout", s=w715, f=w709) -> (s? t:f=w713:string)
                n318 = Format Into String(format string=": %s", initial string=w713, "ON/OFF +5V") -> (resulting string=w710:string)  [unwired: 1 in, 1 out]
                n319 = call "string log (SubVI).vi"("state Name"=w710) -> ()  [unwired: 9 in, 2 out]
              }
              frame condition #1 {
              }
            }
            n320 = To Variant(anything="5V Value") -> (Variant=w705:variant)
            n321 = call "App enquece.vi"("command data"=w705, "command"="MEAS.Turn+5V", "queue in"=w708) -> ("error out"=w707:errorcluster)  [unwired: 7 in, 1 out]
            n322 = Merge Errors(w700, w707) -> (w701:errorcluster)
          }
          event "mux 6-1": Value Change {
            n323 = event-data() -> ()  [unwired: 1 in, 1 out]
            n324 = disable-structure shown="LOGGING==TRUE" {
              disable-tunnel: w723 -> [w751 _]
              frame condition #0 (active) {
                n325 = Empty String/Path?(string/path=w751) -> (empty?=w757:bool)
                n326 = Select(t="Quece timeout", s=w757, f=w751) -> (s? t:f=w755:string)
                n327 = Format Into String(format string=": %s", initial string=w755, "mux6-1") -> (resulting string=w752:string)  [unwired: 1 in, 1 out]
                n328 = call "string log (SubVI).vi"("state Name"=w752) -> ()  [unwired: 9 in, 2 out]
              }
              frame condition #1 {
              }
            }
            n329 = Decrement(x=w720) -> (x-1=w719:i32)
            n330 = Multiply(x=w719, y=6) -> (x*y=w717:i32)
            n331 = case shown="\"mux6_1_channel3_3\"" "mux 6-1 data" {
              tunnel: w717 -> [_ w735 w738 w741 w744 w747 w750]
              tunnel: [0 w733 w736 w739 w742 w745 w748] -> w716
              frame "mux6-1_channel0", Default {
              }
              frame "mux6_1_channel1_3" {
                n332 = Add(x=w735, y=0) -> (x+y=w733:i32)
              }
              frame "mux6_1_channel2_3" {
                n333 = Add(x=w738, y=1) -> (x+y=w736:i32)
              }
              frame "mux6_1_channel3_3" {
                n334 = Add(x=w741, y=2) -> (x+y=w739:i32)
              }
              frame "mux6_1_channel4_3" {
                n335 = Add(x=w744, y=3) -> (x+y=w742:i32)
              }
              frame "mux6_1_channel5_3" {
                n336 = Add(x=w747, y=4) -> (x+y=w745:i32)
              }
              frame "mux6_1_channel6_3" {
                n337 = Add(x=w750, y=5) -> (x+y=w748:i32)
              }
            }
            n338 = To Variant(anything="mux 6-1 data") -> (Variant=w727:variant)
            n339 = call "App enquece.vi"("command data"=w727, "command"="MEAS.mux6_1", "queue in"=w728) -> ("error out"=w726:errorcluster)  [unwired: 7 in, 1 out]
            n340 = Merge Errors(w724, w726) -> (w725:errorcluster)
          }
          event "Mux 10-1": Value Change {
            n341 = event-data() -> ()  [unwired: 1 in, 1 out]
            n342 = disable-structure shown="LOGGING==TRUE" {
              disable-tunnel: w761 -> [w771 _]
              frame condition #0 (active) {
                n343 = Empty String/Path?(string/path=w771) -> (empty?=w777:bool)
                n344 = Select(t="Quece timeout", s=w777, f=w771) -> (s? t:f=w775:string)
                n345 = Format Into String(format string=": %s", initial string=w775, "mux10-1") -> (resulting string=w772:string)  [unwired: 1 in, 1 out]
                n346 = call "string log (SubVI).vi"("state Name"=w772) -> ()  [unwired: 9 in, 2 out]
              }
              frame condition #1 {
              }
            }
            n347 = To Variant(anything="mux 10-1 data") -> (Variant=w766:variant)
            n348 = call "App enquece.vi"("command data"=w766, "command"="MEAS.mux10-1", "queue in"=w769) -> ("error out"=w763:errorcluster)  [unwired: 7 in, 1 out]
            n349 = Merge Errors(w764, w763) -> (w762:errorcluster)
          }
          event "request AC-all": Value Change {
            w784 = T6 {"eMIC 1"={"ACV"=0.0, "ACI"=0.0, "pF"=0.0, "kW"=0.0, "Freq"=0.0, "kvar"=0.0}, "eMIC 2"={"ACV"=0.0, "ACI"=0.0, "pF"=0.0, "kW"=0.0, "Freq"=0.0, "kvar"=0.0}, "eMIC 3"={"ACV"=0.0, "ACI"=0.0, "pF"=0.0, "kW"=0.0, "Freq"=0.0, "kvar"=0.0}, "eMIC 4"={"ACV"=0.0, "ACI"=0.0, "pF"=0.0, "kW"=0.0, "Freq"=0.0, "kvar"=0.0}, "eMIC 5"={"ACV"=0.0, "ACI"=0.0, "pF"=0.0, "kW"=0.0, "Freq"=0.0, "kvar"=0.0}, "eMIC 6"={"ACV"=0.0, "ACI"=0.0, "pF"=0.0, "kW"=0.0, "Freq"=0.0, "kvar"=0.0}}  # eMICs cluster
            n350 = event-data() -> ()  [unwired: 1 in, 1 out]
            n351 = disable-structure shown="LOGGING==TRUE" {
              disable-tunnel: w785 -> [w791 _]
              frame condition #0 (active) {
                n352 = Empty String/Path?(string/path=w791) -> (empty?=w798:bool)
                n353 = Select(t="Quece timeout", s=w798, f=w791) -> (s? t:f=w796:string)
                n354 = Format Into String(format string=": %s", initial string=w796, "request AC") -> (resulting string=w793:string)  [unwired: 1 in, 1 out]
                n355 = call "string log (SubVI).vi"("Enum(log)"=enum16{"Init", "Log", "Read"}."Log" ("Enum"), "state Name"=w793) -> ()  [unwired: 8 in, 2 out]
              }
              frame condition #1 {
              }
            }
            n356 = call "FGV wait for 6 eMICs.vi"("Enum"=enum16{"Init", "count"}."Init") -> ("error out"=w781:errorcluster)  [unwired: 8 in, 2 out]
            n357 = call "App enquece.vi"("error in (no error)"=w781, "command"="MEAS.requestAC", "queue in"=w790) -> ("error out"=w786:errorcluster)  [unwired: 7 in, 1 out]
            n358 = Merge Errors(w787, w786) -> (w783:errorcluster)
          }
          event User Event {
            n359 = event-data() -> ("Module ID"=w809:i32, "Array"=w824:T23[])  [unwired: 1 in]
            n360 = Variant To Data(type=0, Variant=w805) -> (data=w803:i32)  [unwired: 1 in, 1 out]
            n361 = for {
              tunnel: w824 -> [w886] mode=indexing
              shift-right: [w882] -> w800
              shift-left: T5 {"ACV"=0.0, "ACI"=0.0, "pF"=0.0, "kW"=0.0, "Freq"=0.0, "kvar"=0.0} ("eMIC response") -> [w884]
              n362 = Unbundle By Name(w886) -> ("float"=w883:dbl, "Name"=w885:string)
              n363 = case shown="\"kW\"" w885 {
                tunnel: w884 -> [w887 w890 w893 w896 w899 w902 w905]
                tunnel: w883 -> [_ w888 w891 w894 w898 w900 w904]
                tunnel: [w887 w889 w892 w895 w897 w901 w903] -> w882
                frame "False", Default {
                }
                frame "ACI" {
                  n364 = Bundle By Name(cluster=w890, "ACI"=w888) -> (w889:T5)
                }
                frame "kW" {
                  n365 = Bundle By Name(cluster=w893, "kW"=w891) -> (w892:T5)
                }
                frame "PF" {
                  n366 = Bundle By Name(cluster=w896, "pF"=w894) -> (w895:T5)
                }
                frame "ACV" {
                  n367 = Bundle By Name(cluster=w899, "ACV"=w898) -> (w897:T5)
                }
                frame "Freq" {
                  n368 = Bundle By Name(cluster=w902, "Freq"=w900) -> (w901:T5)
                }
                frame "kvar" {
                  n369 = Bundle By Name(cluster=w905, "kvar"=w904) -> (w903:T5)
                }
              }
            }
            n370 = disable-structure shown="LOGGING==TRUE" {
              disable-tunnel: w810 -> [w860 _]
              disable-tunnel: w809 -> [w856 _]
              frame condition #0 (active) {
                n371 = Empty String/Path?(string/path=w860) -> (empty?=w862:bool)
                n372 = Select(t="Quece timeout", s=w862, f=w860) -> (s? t:f=w859:string)
                n373 = Format Into String(format string=":%s %d", initial string=w859, "CE14  data response", w856) -> (resulting string=w855:string)  [unwired: 1 in, 1 out]
                n374 = call "string log (SubVI).vi"("state Name"=w855) -> ()  [unwired: 9 in, 2 out]
              }
              frame condition #1 {
              }
            }
            n375 = call "eMIC_calibration.vi"("eMIC data in"=w800) -> ("eMIC data out"=w799:T5)  [unwired: 10 in]
            n376 = case shown="6" w809 {
              tunnel: [w863 w865 w868 w871 w874 w877 w880] -> w815
              tunnel: w816 -> [w863 w866 w869 w872 w875 w878 w881]
              tunnel: w799 -> [_ w864 w867 w870 w873 w876 w879]
              frame 0, Default {
              }
              frame 1 {
                n377 = Bundle By Name(cluster=w866, "eMIC 1"=w864) -> (w865:T6)
              }
              frame 2 {
                n378 = Bundle By Name(cluster=w869, "eMIC 2"=w867) -> (w868:T6)
              }
              frame 3 {
                n379 = Bundle By Name(cluster=w872, "eMIC 3"=w870) -> (w871:T6)
              }
              frame 4 {
                n380 = Bundle By Name(cluster=w875, "eMIC 4"=w873) -> (w874:T6)
              }
              frame 5 {
                n381 = Bundle By Name(cluster=w878, "eMIC 5"=w876) -> (w877:T6)
              }
              frame 6 {
                n382 = Bundle By Name(cluster=w881, "eMIC 6"=w879) -> (w880:T6)
              }
            }
            n383 = case shown="0" w803 {
              tunnel: w815 -> [w832 w850]
              tunnel: w814 -> [w831 _]
              tunnel: [w829 w848] -> w811
              tunnel: w807 -> [w828 w854]
              tunnel: [w827 w854] -> w806
              tunnel: w802 -> [w826 w851]
              tunnel: [w826 w851] -> w801
              frame 0 {
                n384 = call "FGV wait for 6 eMICs.vi"("Enum"=enum16{"Init", "count"}."count") -> ("error out"=w830:errorcluster, "wait done"=w833:bool)  [unwired: 8 in, 1 out]
                "AC  Completed" <- w833
                n385 = case shown="True" w833 {
                  tunnel: w832 -> [_ w843]
                  tunnel: w828 -> [w835 w841]
                  tunnel: w831 -> [w840 _]
                  tunnel: w830 -> [w837 w845]
                  tunnel: [w836 w844] -> w829
                  tunnel: [w835 w841] -> w827
                  frame False {
                    n386 = call "App enquece.vi"("Priority Enquece"=TRUE, "error in (no error)"=w837, "command"="Apps.WaitForEvent", "queue in"=w840) -> ("error out"=w836:errorcluster)  [unwired: 6 in, 1 out]
                  }
                  frame True {
                    n387 = To Variant(anything=w843) -> (Variant=w842:variant)
                    n388 = call "FGV Driver Data.vi"("DUT channel (1-11)"=w841, "Mode"=DUT_data_Mode."AC parameter", "error in (no error)"=w845, "FGV enum(Read)"=FGV_DRV_data."Write" ("FGV DRV data enum"), "data"=w842) -> ("error out"=w844:errorcluster)  [unwired: 3 in, 3 out]
                  }
                }
              }
              frame 1, Default {
                n389 = To Variant(anything=w850) -> (Variant=w849:variant)
                n390 = call "FGV Driver Data.vi"("Mode"=DUT_data_Mode."AC parameter 1", "DUT index(1-60)"=w851, "FGV enum(Read)"=FGV_DRV_data."Write", "data"=w849) -> ("error out"=w848:errorcluster)  [unwired: 4 in, 3 out]
              }
            }
            n391 = Unbundle By Name(w815) -> ("eMIC 1"=→"eMIC 1":T5, "eMIC 2"=→"eMIC 2":T5, "eMIC 3"=→"eMIC 3":T5, "eMIC 4"=→"eMIC 4":T5, "eMIC 5"=→"eMIC 5":T5, "eMIC 6"=→"eMIC 6":T5)
            n392 = Merge Errors(w812, w811) -> (w813:errorcluster)
          }
          event User Event {
            n393 = event-data() -> ("Init?"=w919:bool, "Module ID"=w906:i32)  [unwired: 1 in]
            "Module ID" <- w906
            "AC Measure Module" <- w919
            n394 = disable-structure shown="LOGGING==TRUE" {
              disable-tunnel: w921 -> [w940 _]
              disable-tunnel: w906 -> [w936 _]
              frame condition #0 (active) {
                n395 = Empty String/Path?(string/path=w940) -> (empty?=w942:bool)
                n396 = Select(t="Quece timeout", s=w942, f=w940) -> (s? t:f=w939:string)
                n397 = Format Into String(format string=":%s %d", initial string=w939, "CE14 Did  it", w936) -> (resulting string=w935:string)  [unwired: 1 in, 1 out]
                n398 = call "string log (SubVI).vi"("state Name"=w935) -> ()  [unwired: 9 in, 2 out]
              }
              frame condition #1 {
              }
            }
            n399 = Decrement(x=w906) -> (x-1=w920:i32)
            n400 = Initialize Array(FALSE, 6 ("dimension size")) -> (w915:bool[])
            n401 = feedback #2(w915) -> (w916:bool[])
            n402 = Replace Array Subset(array=w916, new element=w919, index=w920) -> (w914:bool[])
            "CE14  Module did it" <- w914
            n403 = feedback-in #2(w914) -> ()
            n404 = And Array Elements(Boolean array=w914) -> (logical AND=w913:bool)
            n405 = case shown="True" w913 {
              tunnel: w912 -> [_ w928]
              tunnel: [_ w927] -> w911
              frame False {
              }
              frame True {
                n406 = flat-sequence {
                  tunnel: [w930] -> w929
                  tunnel: w928 -> [w930]
                  tunnel: w929 -> [w933]
                  tunnel: [w932] -> w927
                  frame #0 {
                    n407 = Wait (ms)(milliseconds to wait=u32 500) -> ()  [unwired: 1 out]
                  }
                  frame #1 {
                    n408 = call "App enquece.vi"("command"="MEAS.Read EMIC connected", "queue in"=w933) -> ("error out"=w932:errorcluster)  [unwired: 8 in, 1 out]
                  }
                }
              }
            }
            n409 = control-ref of="Select CE14 eMIC Module Instance"() -> (w926:refnum<vi>)
            n410 = call "Update Select Module Ring.vi"("Select Module Ring Ref"=w926) -> ("error out"=w910:errorcluster)  [unwired: 8 in, 2 out]
            n411 = Merge Errors(w922, w911, w910) -> (w923:errorcluster)
          }
          event "Shorted Circuits Test": Value Change {
            n412 = event-data() -> ()  [unwired: 1 in, 1 out]
            n413 = disable-structure shown="Enabled" {
              frame Enabled {
                n414 = Initialize Array(FALSE, 6 ("dimension size"), 10 ("dimension size")) -> (w954:bool[][])
                n415 = local write "Short DRV"(w954) -> ()
              }
              frame Disabled {
              }
            }
            n416 = Build Array("Test Shorted Circuits") -> (w948:string[])
            n417 = for {
              tunnel: [w960] -> w949 mode=indexing
              tunnel: w948 -> [w959] mode=indexing
              tunnel: w947 -> [w958]
